vi "Задание_АБ_система ask +.vi"() -> ()   [LabVIEW 2017]
uses:
  <vilib>/Analysis/baseanly.llb/Mean (DBL).vi
  <vilib>/Waveform/DWDTOps.llb/DWDT Analog to Digital.vi
  <vilib>/gmath/statdist.llb/Normal Random.vi
  <vilib>/gmath/NI_Gmath.lvlib
  <vilib>/Analysis/NI_AALBase.lvlib
panel:
  out "Вектор ошибки неправильно":ext[](array[numeric])
  out "Размер сообщения":i32
  out "output bit stream":i8[](array[numeric]) caption="Демодулированный ASK"
  out "Digital Waveform Graph 3":digitalwaveform(graph)
  in  "pulse shaping filter (none) 2":T1(ring) caption="pulse shaping filter (none)"
  in  "passband bandwidth (Hz)":dbl format="%.2p"
  in  "carrier frequency (Hz) 2":dbl caption="carrier frequency (Hz)" min=-0.5 max=0.5 format="%.2p"
  out "Rs":dbl
  in  "carrier frequency (Hz)":dbl min=-0.5 max=0.5 format="%.2f"
  in  "pulse shaping filter (none)":T1(ring)
  in  "Ts":dbl
  in  "Fs":dbl
  out "Сигнал в канале":waveform(dbl)[](graph)
  out "Декодированное исходное":dbl[](array[numeric])
  out "Декодированное сообщение 2":dbl[](array[numeric])
  out "Размер окна с паузами":i32
  out "output array":dbl[](array[numeric])
  in  "Кол-во копий":i32=5
  out "Подготовленный к отправке мажоритарный код":dbl[][](array[numeric])
  out "Демодулированный сигнал 2":i16[](graph)
  out "Демодулированный сигнал (заполнение)":i16[](array[numeric])
  in  "Пороговое значение 2":dbl
  out "Среднее значение":dbl[](array[numeric])
  out "Шум на основе распределения Рэлея":dbl[](graph)
  out "Демодулированный и отфильтрованный сигнал":dbl[](graph)
  in  "Нижняя частота среза":dbl
  in  "Порядок фильтра":i64(slide) scale=0.0..20.0
  in  "Переменная floor(x/y)":i32
  out "Модулирующий сигнал":dbl[](graph)
  out "Частотно модулированный цифровой сигнал":dbl[](graph)
  in  "см. 1.2 Циклов в секунду":i32(slide) scale=4.0..50.0
  in  "Сколько битов брать":i32=4
  out "Радио сигнал с паузами":dbl[](graph)
  in  "Кол-во выборок":i32=400
  out "Массив с паузами":dbl[](array[numeric])
  in  "Количество бит":i32=8
  out "Вырезка из массива":dbl[](array[numeric])
  out "Биты на выходе 1":dbl[](array[numeric])
  # "Демодуляция"
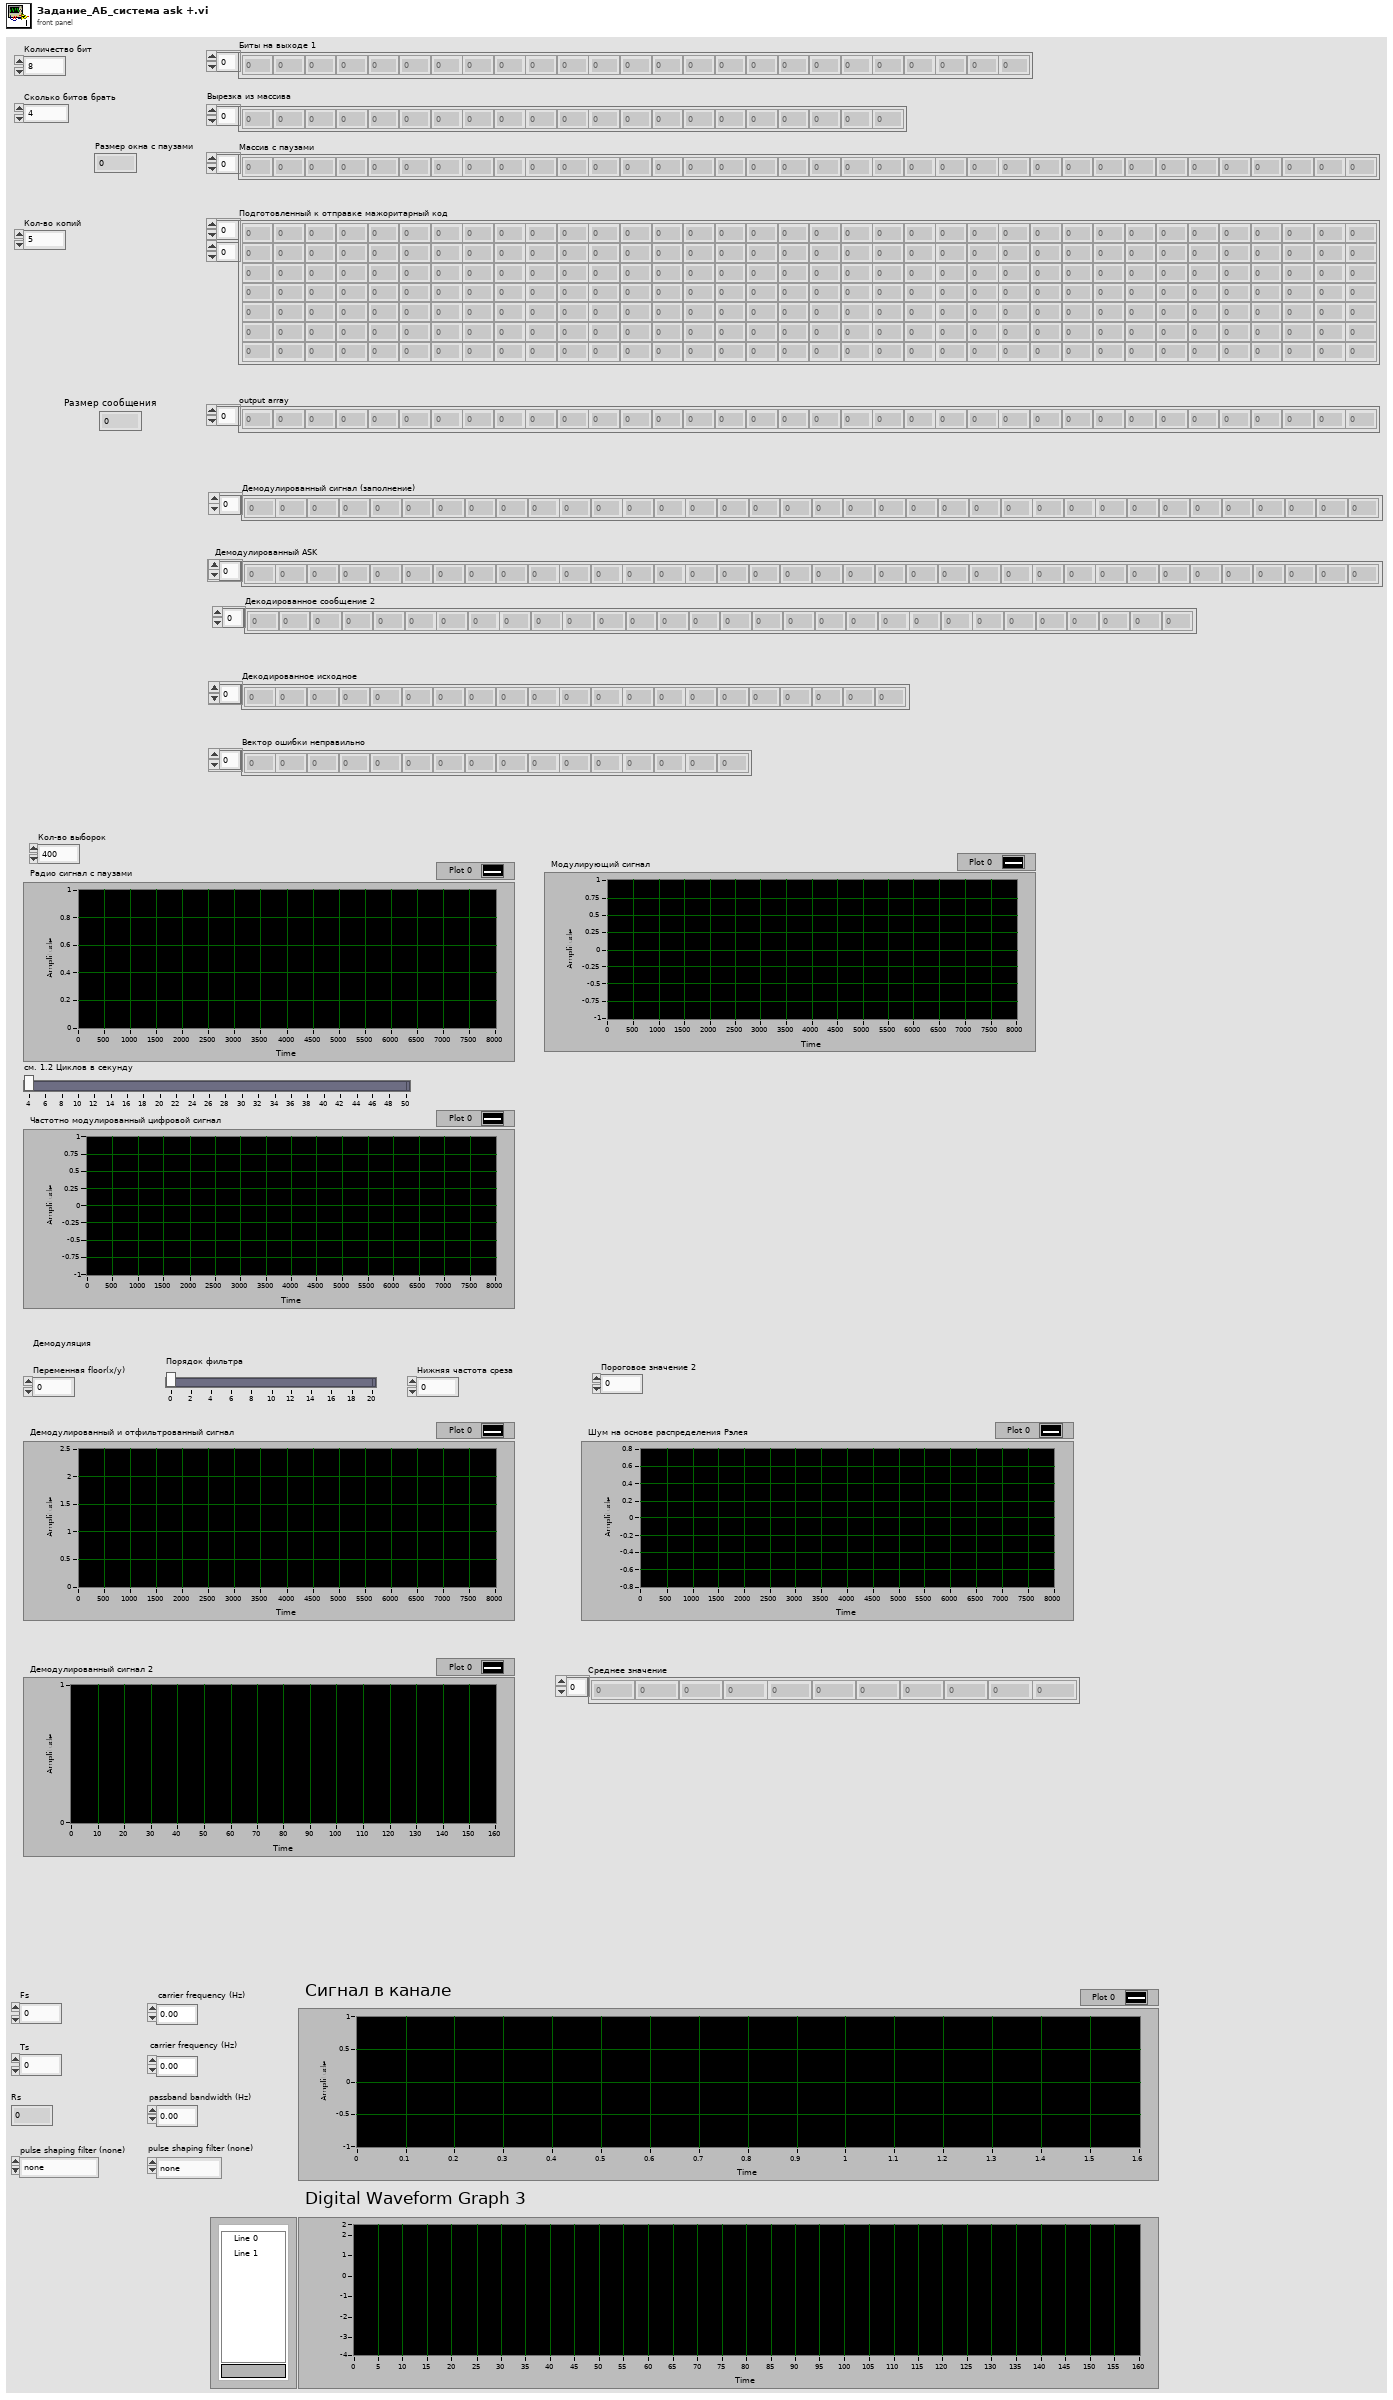
[diagram p1: front panel]
types:
  T1 = enum16{"none", "Raised Cosine", "Root Raised Cos", "Gaussian"}
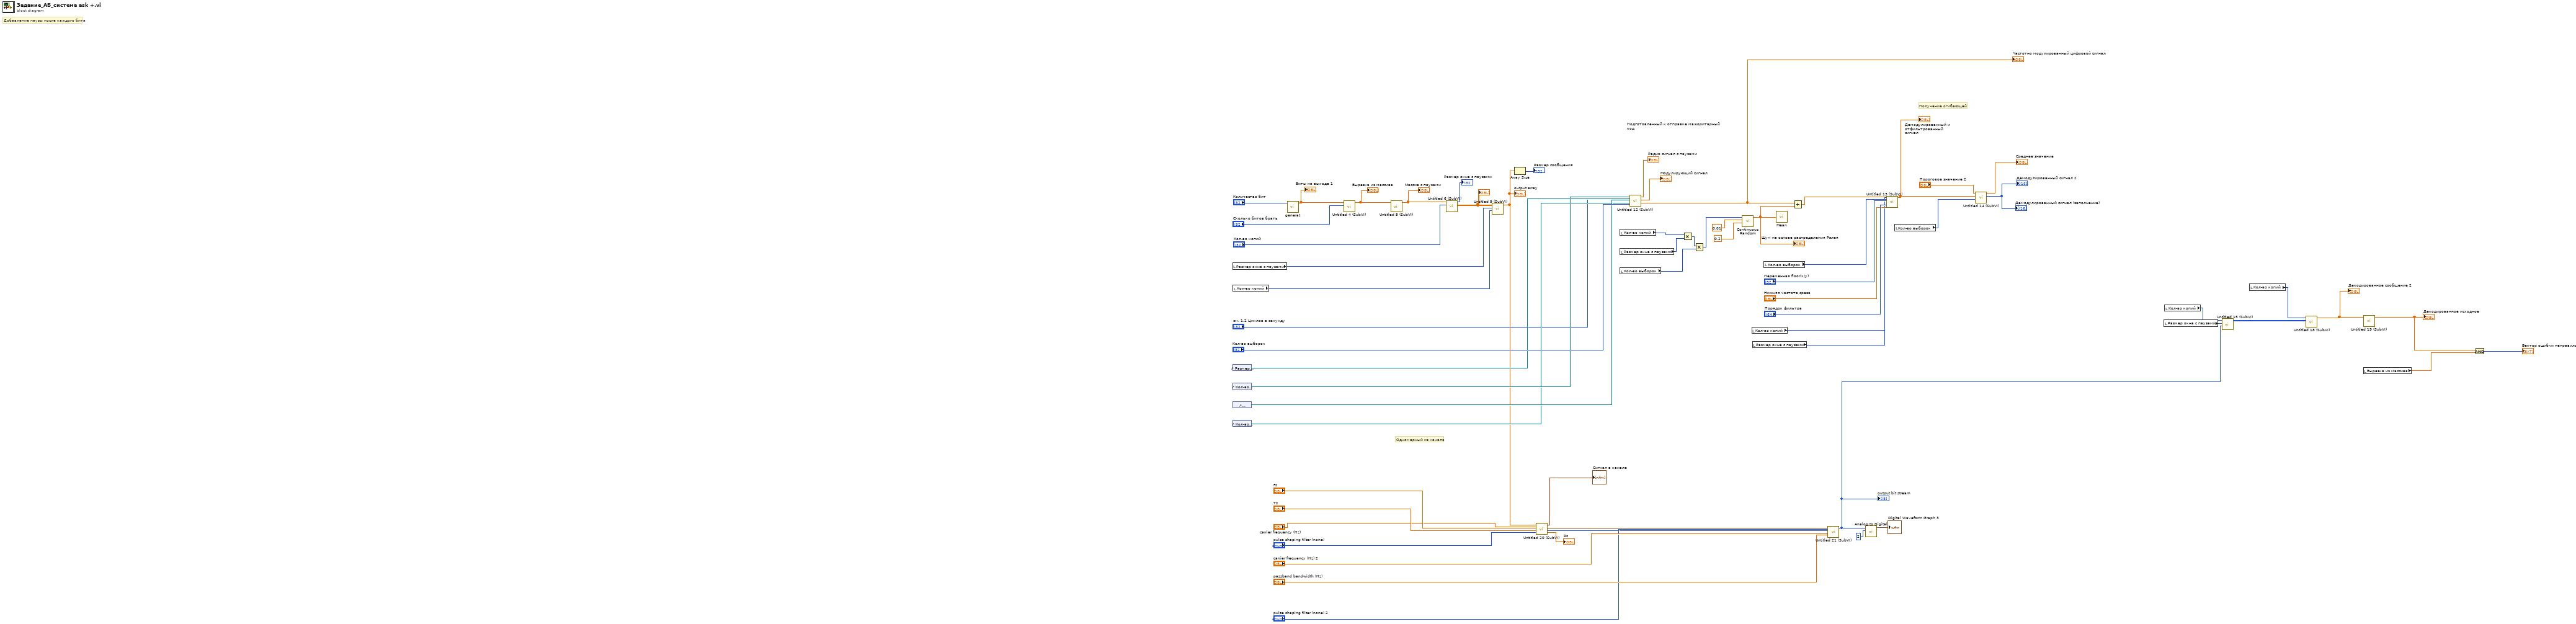
[diagram p0: block diagram]
diagram:
  # "Одномерный из канала"
  # "Получение огибающей"
  # "Добавление паузы после каждого бита"
  n1 = local read "Размер окна с паузами"() -> (w43:i32)
  n2 = control-ref of="Размер окна с паузами"() -> (w13:refnum<vi>)
  n3 = control-ref of="Кол-во выборок"() -> (w14:refnum<vi>)
  n4 = control-ref of="Переменная floor(x/y)"() -> (w12:refnum<vi>)
  n5 = control-ref of="Кол-во копий"() -> (w11:refnum<vi>)
  n6 = local read "Кол-во копий"() -> (w42:i32)
  n7 = call "generat.vi"("Количество бит"="Количество бит") -> ("Array"=w8:dbl[])  [unwired: 10 in]
  "Биты на выходе 1" <- w8
  n8 = call "Untitled 4 (SubVI).vi"("Сколько битов брать"="Сколько битов брать", "Array in"=w8) -> ("Array out"=w61:dbl[])  [unwired: 9 in]
  "Вырезка из массива" <- w61
  n9 = call "Untitled 5 (SubVI).vi"("Array in"=w61) -> ("Array"=w38:dbl[])  [unwired: 10 in]
  "Массив с паузами" <- w38
  n10 = call "Untitled 6 (SubVI).vi"("Кол-во копий"="Кол-во копий", "Array"=w38) -> ("см. 1.5"=w36:dbl[][], "Numeric"=→"Размер окна с паузами":i32)  [unwired: 8 in]
  "Подготовленный к отправке мажоритарный код" <- w36
  n11 = call "Untitled 9 (SubVI).vi"("Кол-во копий"=w42, "Размер окна с паузами"=w43, "см. 1.5 in"=w36) -> ("см. 1.5 out"=w5:dbl[])  [unwired: 8 in]
  "output array" <- w5
  n12 = Array Size(array=w5) -> (size(s)=→"Размер сообщения":i32)
  n13 = call "Untitled 20 (SubVI).vi"("pulse shaping filter (none)"="pulse shaping filter (none)", "carrier frequency (Hz)"="carrier frequency (Hz)", "Ts"="Ts", "Fs"="Fs", "см. 1.5 in"=w5) -> ("Numeric"=w20:i32, "passband waveform"=w24:waveform(dbl), "Array"=→"Сигнал в канале":waveform(dbl)[], "Rs"=→"Rs":dbl)  [unwired: 3 in]
  n14 = local read "Кол-во копий"() -> (w52:i32)
  n15 = local read "Размер окна с паузами"() -> (w51:i32)
  n16 = local read "Кол-во выборок"() -> (w33:i32)
  n17 = call "Untitled 12 (SubVI).vi"("см. 1.2 Циклов в секунду"="см. 1.2 Циклов в секунду", "Кол-во выборок"="Кол-во выборок", "reference in"=w13, "reference 4"=w11, "reference 3"=w12, "Digital in"=w14) -> ("Array"=w49:dbl[], "Модулирующий сигнал"=→"Модулирующий сигнал":dbl[], "Pulse Pattern"=→"Радио сигнал с паузами":dbl[])  [unwired: 3 in]
  "Частотно модулированный цифровой сигнал" <- w49
  n18 = Multiply(x=w52, y=w51) -> (x*y=w35:i32)
  n19 = Multiply(x=w35, y=w33) -> (x*y=w34:i32)
  n20 = call-poly <vilib>:"Continuous Random.vi"("std"=0.2 ("b"), "mean"=0.01 ("x"), "samples"=w34) -> ("normal random data"=w50:dbl[])  [unwired: 7 in, 1 out]
  "Шум на основе распределения Рэлея" <- w50
  n21 = local read "Кол-во копий"() -> (w32:i32)
  n22 = local read "Размер окна с паузами"() -> (w55:i32)
  n23 = local read "Кол-во выборок"() -> (w56:i32)
  n24 = call-poly <vilib>:"Mean.vi"("X"=w50) -> ()  [unwired: 2 out]
  n25 = Add(x=w49, y=w50) -> (x+y=w48:dbl[])
  n26 = call "Untitled 21 (SubVI).vi"("passband bandwidth (Hz)"="passband bandwidth (Hz)", "pulse shaping filter (none) in"="pulse shaping filter (none) 2", "carrier frequency (Hz) in"="carrier frequency (Hz) 2", "Numeric"=w20, "passband waveform"=w24) -> ("output bit stream"=w16:i8[])  [unwired: 6 in]
  "output bit stream" <- w16
  n27 = call-poly <vilib>:"Analog to Digital.vi"("resolution (16 bit)"=2, "analog waveform"=w16) -> ("digital waveform"=→"Digital Waveform Graph 3":digitalwaveform)  [unwired: 6 in, 3 out]
  n28 = call "Untitled 13 (SubVI).vi"("Порядок фильтра"="Порядок фильтра", "Array"=w48, "Нижняя частота среза"="Нижняя частота среза", "Кол-во выборок"=w56, "Переменная floor(x/y)"="Переменная floor(x/y)", "Кол-во копий"=w32, "Размер окна с паузами"=w55) -> ("Filtered X"=w47:dbl[])  [unwired: 4 in]
  "Демодулированный и отфильтрованный сигнал" <- w47
  n29 = local read "Кол-во выборок"() -> (w46:i32)
  n30 = call "Untitled 14 (SubVI).vi"("Кол-во выборок"=w46, "Filtered X"=w47, "Пороговое значение in"="Пороговое значение 2") -> ("Array"=→"Демодулированный сигнал (заполнение)" →"Демодулированный сигнал 2":i16[], "Array 2"=→"Среднее значение":dbl[])  [unwired: 7 in]
  n31 = local read "Размер окна с паузами"() -> (w39:i32)
  n32 = local read "Кол-во копий"() -> (w31:i32)
  n33 = call "Untitled 15 (SubVI).vi"("output bit stream"=w16, "Размер окна с паузами"=w39, "Кол-во копий"=w31) -> ("Array"=w40:i8[][])  [unwired: 8 in]
  n34 = local read "Кол-во копий"() -> (w41:i32)
  n35 = call "Untitled 18 (SubVI).vi"("Array in"=w40, "Кол-во копий"=w41) -> ("Array out"=w30:dbl[])  [unwired: 9 in]
  "Декодированное сообщение 2" <- w30
  n36 = local read "Вырезка из массива"() -> (w2:dbl[])
  n37 = call "Untitled 19 (SubVI).vi"("Array in"=w30) -> ("Array"=w3:dbl[])  [unwired: 10 in]
  "Декодированное исходное" <- w3
  n38 = And(x=w3, y=w2) -> (x .and. y?=→"Вектор ошибки неправильно":i32[])
